vi "fill list from array.vi"(1 "channel  names":string[](array[string])) -> (0 "channel list out":i32[](listbox)=[4])   [LabVIEW 2013]
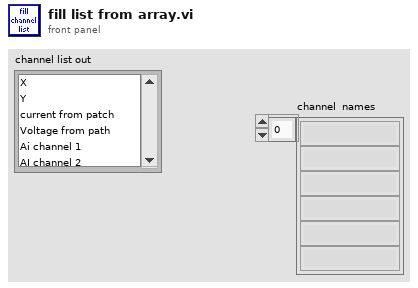
[diagram p1: front panel]
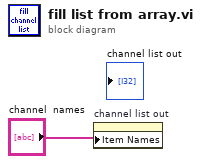
[diagram p0: block diagram]
diagram:
  n1 = property on="channel list out" class="LstBox (strict)"("Item Names"="channel  names") -> ()  [unwired: 2 in, 2 out]
